vi "GUI_Frog_HPD_imagetested2.vi"() -> ()   [LabVIEW 2013]
uses:
  Shared/GUI_Template/GUI_master/tcp_new_data_event.ctl
  Shared/GUI_Template/GUI_master/tcp new data cluster.ctl
panel:
  in  "triggermode::1":bool caption="Blank Button"
  out "retrievedFrogTrace::1":T1(plugin-control) caption="Retrieved Frog Trace"
  out "frogTrace::1":T1(plugin-control) caption="FROG Trace"
  in  "insert tag":bool=TRUE
  in  "stop":bool
  in  "GUIdevice 1":string="FrogHPD"
  out "tcp data event":T2
  out "error IO 2":errorcluster
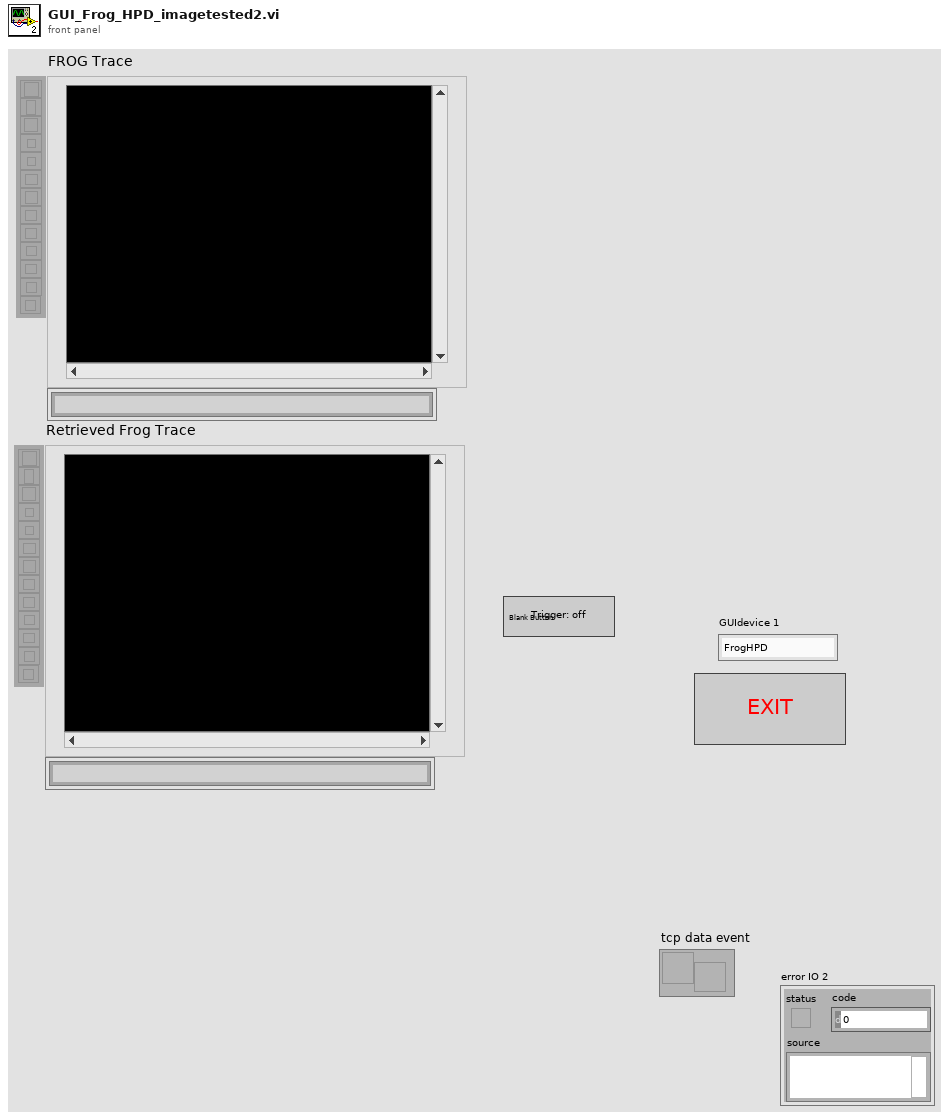
[diagram p1: front panel]
types:
  T1 = typedef "IMAQ Image.ctl" = refnum<image>
  T2 = typedef "tcp_new_data_event.ctl" = refnum<user-event>
  T3 = typedef "Image Type" = u32
  T4 = typedef "tcp new data cluster.ctl" = cluster{"EventEnum":enum16{"new data", "connection status update"}, "Device name":string}
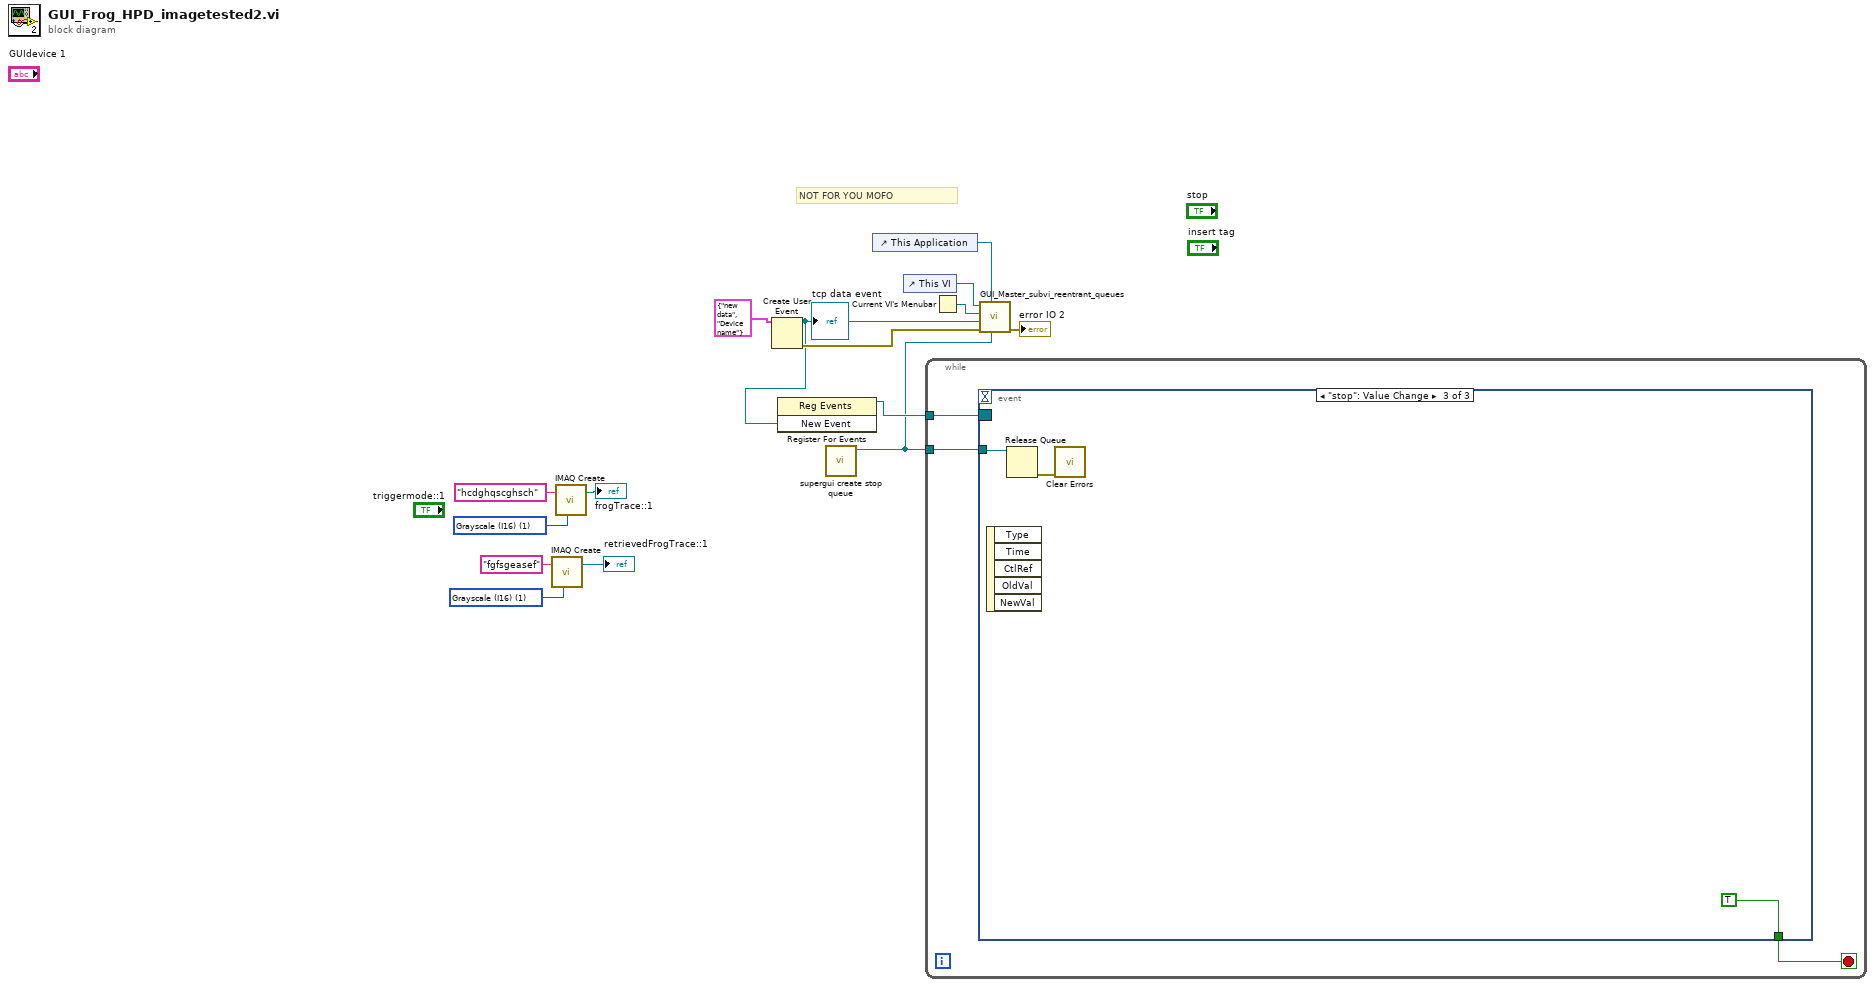
[diagram p0: block diagram]
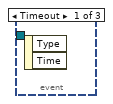
[diagram p2: hidden frame]
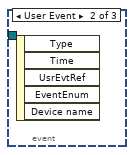
[diagram p3: hidden frame]
diagram:
  w4 = T3 1 items=["Grayscale (U8)", "Grayscale (I16)", "Grayscale (SGL)", "Complex (CSG)", "RGB (U32)", "HSL (U32)", "RGB (U64)", "Grayscale (U16)"] ("Image Type")
  w6 = T3 1 items=["Grayscale (U8)", "Grayscale (I16)", "Grayscale (SGL)", "Complex (CSG)", "RGB (U32)", "HSL (U32)", "RGB (U64)", "Grayscale (U16)"] ("Image Type")
  # "NOT FOR YOU MOFO"
  n1 = call "IMAQ Create"("Image Name"="fgfsgeasef", "Image Type"=w4) -> ("New Image"=→"retrievedFrogTrace::1":T1)  [unwired: 3 in, 1 out]
  n2 = call "IMAQ Create"("Image Name"="hcdghqscghsch", "Image Type"=w6) -> ("New Image"=→"frogTrace::1":T1)  [unwired: 3 in, 1 out]
  n3 = Create User Event(user event datatype=T4 {"EventEnum"=enum."new data", "Device name"="Device name"} ("New Event")) -> (user event=w9:refnum<user-event>, error out=w11:errorcluster)  [unwired: 1 in]
  "tcp data event" <- w9
  n4 = register-events(w9) -> (reference out=w8:refnum<event-registration>)  [unwired: 2 in, 1 out]
  n5 = call "supergui create stop queue.vi"() -> ("STOP Queue out"=w1:refnum<queue>)  [unwired: 11 in]
  n6 = control-ref of="This Application"() -> (w10:refnum<vi>)
  n7 = control-ref of="This VI"() -> (w14:refnum<vi>)
  n8 = while {
    tunnel: w8 -> [w17]
    tunnel: w1 -> [w16]
    stop <- w18 stop-if-true
    n9 = event shown="[2] \"stop\": Value Change" {
      selector: w17 -> [_ _ _]
      dyn-events: _ -> [_ _ _]
      timeout: _ -> [_ _ _]
      tunnel: [_ _ TRUE] -> w18
      tunnel: w16 -> [_ _ w20]
      event Timeout {
        n10 = event-data() -> ()  [unwired: 1 in, 2 out]
      }
      event User Event {
        n11 = event-data() -> ()  [unwired: 1 in, 5 out]
      }
      event "stop": Value Change {
        n12 = event-data() -> ()  [unwired: 1 in, 5 out]
        n13 = Release Queue(queue=w20) -> (error out=w19:errorcluster)  [unwired: 2 in, 2 out]
        n14 = call <vilib>:"Clear Errors.vi"("error in (no error)"=w19) -> ()  [unwired: 6 in, 1 out]
      }
    }
  }
  n15 = Current VI's Menubar() -> (w13:refnum<k9>)
  n16 = call "GUI_Master_subvi_reentrant_queues.vi"("STOP Queue in"=w1, "This Application"=w10, "error in (no error)"=w11, "tcp data event"=w9, "Caller menu reference"=w13, "Caller VI ref"=w14) -> ("error out"=→"error IO 2":errorcluster)  [unwired: 5 in]
